vi "Write Roles.vi"(8 "error in (no error)":errorcluster, 10 "Roles":T1, 11 "KeeperPassToStrikerPlay in":refnum<class "KeeperPassToStrikerPlay.lvclass">) -> (0 "error out":errorcluster, 3 "KeeperPassToStrikerPlay out":refnum<class "KeeperPassToStrikerPlay.lvclass">)   [LabVIEW 2024, in "KeeperPassToStrikerPlay.lvclass"]
uses:
  KeeperPassToStrikerPlay.lvclass
  WaitPassRole_class/WaitPassRole.lvclass
  FollowAttackerRole_class/FollowAttackerRole.lvclass
  KeeperPassToStrikerPlay.lvclass/KeeperPassToStrikerPlay.ctl
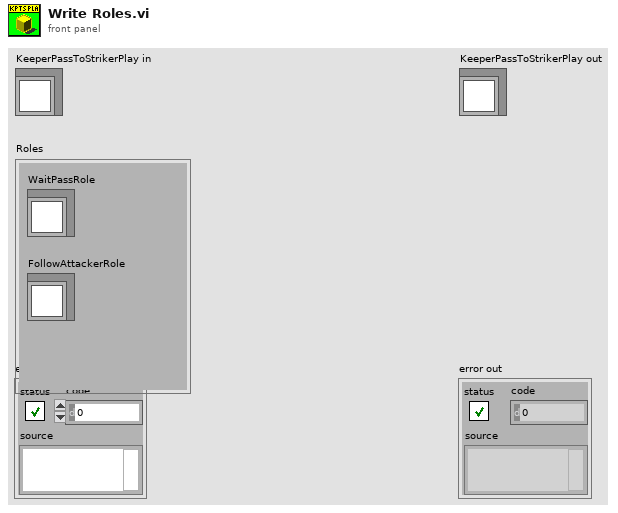
[diagram p1: front panel]
types:
  T1 = cluster{"WaitPassRole":refnum<class "WaitPassRole.lvclass">, "FollowAttackerRole":refnum<class "FollowAttackerRole.lvclass">}
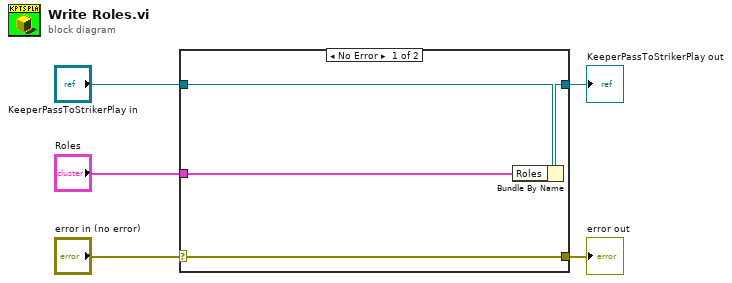
[diagram p0: block diagram]
diagram:
  n1 = case shown="No Error" "error in (no error)" {
    selector: "error in (no error)" -> [w9 w10]
    tunnel: [w9 w10] -> w4
    tunnel: [w7 w11] -> w2
    tunnel: "KeeperPassToStrikerPlay in" -> [w8 w11]
    tunnel: "Roles" -> [w6 _]
    frame No Error {
      n2 = Bundle By Name(cluster=w8, "Roles"=w6) -> (w7:refnum<class "KeeperPassToStrikerPlay.lvclass">)
    }
    frame Error {
    }
  }
  "error out" <- w4
  "KeeperPassToStrikerPlay out" <- w2
